vi "Destroy.vi"(8 "error in (no error)":errorcluster, 11 "Event Registration Refnum":refnum<event-registration>) -> (0 "error out":errorcluster)   [LabVIEW 2017, in "WebServiceImporter.lvlib" / "Main Panel.lvlib" / "Input Info.lvlib" / "Events.lvlib"]
uses:
  <vilib>/Platform/WebService/Main Panel/Pages/Input Info/Events/Events.lvlib
  <vilib>/Platform/WebService/Main Panel/Pages/Authentication/Events/Events.lvlib
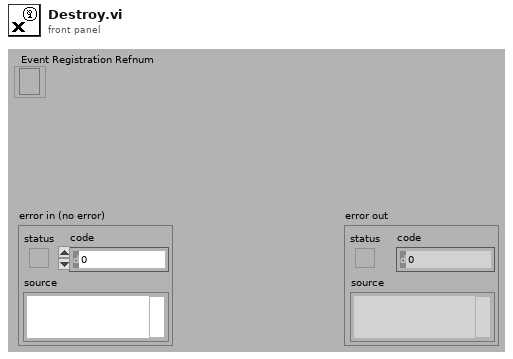
[diagram p1: front panel]
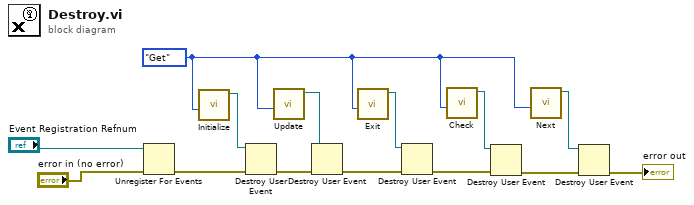
[diagram p0: block diagram]
diagram:
  w4 = enum16{"Get", "Set"}."Get" ("Operation")
  n1 = Unregister For Events(event registration refnum="Event Registration Refnum", error in="error in (no error)") -> (error out=w13:errorcluster)
  n2 = call <vilib>:"Initialize.vi"("Operation"=w4) -> ("user event (out)"=w12:refnum<user-event>)  [unwired: 10 in]
  n3 = Destroy User Event(user event=w12, error in=w13) -> (error out=w7:errorcluster)
  n4 = call <vilib>:"Update.vi"("Operation"=w4) -> ("user event (out)"=w5:refnum<user-event>)  [unwired: 9 in, 1 out]
  n5 = Destroy User Event(user event=w5, error in=w7) -> (error out=w6:errorcluster)
  n6 = call <vilib>:"Exit.vi"("Operation"=w4) -> ("user event (out)"=w11:refnum<user-event>)  [unwired: 9 in, 1 out]
  n7 = Destroy User Event(user event=w11, error in=w6) -> (error out=w10:errorcluster)
  n8 = call <vilib>:"Check.vi"("Operation"=w4) -> ("user event (out)"=w9:refnum<user-event>)  [unwired: 9 in, 1 out]
  n9 = Destroy User Event(user event=w9, error in=w10) -> (error out=w2:errorcluster)
  n10 = call <vilib>:"Next.vi"("Operation"=w4) -> ("user event (out)"=w3:refnum<user-event>)  [unwired: 10 in]
  n11 = Destroy User Event(user event=w3, error in=w2) -> (error out=→"error out":errorcluster)
